vi "Total Nr instrument control to share.vi"() -> ()   [LabVIEW 2018]
panel:
  in  "MFC Max flow (ccm)":cluster{"MFC1":dbl, "MFC2":dbl}={"MFC1"=10000.0, "MFC2"=5000.0}
  out "NOx":cluster{"NO":dbl, "NO2":dbl, "NOx":dbl}(graph)
  out "NO2":dbl format="%#_13g"
  out "NOx":dbl format="%#_13g"
  out "NO":dbl format="%#_13g"
  out "MFC2":dbl format="%#_13g"
  in  "Cluster 2":cluster{"NOx":dbl, "NO":dbl, "NO2":dbl}
  out "Current reading (ppb)":cluster{"NO":dbl, "NOx":dbl, "NO2":dbl}
  in  "Start  Cal":bool
  out "Cal Running time (min)":sgl format="%#_3g"
  in  "read names":T1={"MFC1"="AIN0", "MFC2"="AIN1", "NO"="AIN2", "NOx"="AIN3", "NO2"="AIN5"}
  in  "write names":cluster{"MFC1":string, "MFC2":string}={"MFC1"="TDAC0", "MFC2"="TDAC1"}
  out "MFC flow (ccm)":cluster{"MFC1":dbl, "MFC2":dbl}
  in  "MFC setpoint (ccm)":cluster{"MFC1":dbl, "MFC2":dbl}={"MFC1"=1000.0, "MFC2"=0.0}
  out "valve 4":bool
  out "V4 loop no.":i32
  out "4":dbl
  in  "DIO names":T2={"DIO1"="EIO0", "DIO2"="EIO1", "DIO3"="EIO2", "DIO4"="EIO3", "DIO5"="EIO4", "DIO6"="EIO5"}
  out "Denuder\nTotal Nr":bool
  out "V3 loop no.":i32
  out "3":dbl
  out "Device Temp (K)":dbl[](array[numeric]) format="%.6f"
  in  "Valve switch":T3
  out "ConnectionType Out":i32
  out "DeviceType Out\n7 = T7":i32
  in  "Identifier":string="LJM_idANY"
  in  "ConnectionType":string="LJM_ctANY"
  in  "DeviceType":string="LJM_dtANY"
  out "Error String":string
  out "error out":errorcluster
  out "Total running \ntime (min)":dbl format="%#_3g"
  out "?":cluster{"1":dbl, dbl, dbl}(graph)
  out "1":dbl format="%#_13g"
  in  "Time interval (min)":T4={"Inlet HONO/Total Nr\nValve 1 "=10.0, "HONO/Nox\nValve 2"=5.0, "Total Nr Gas/NH3\nValve 3"=5.0, "valve 5"=1.0, "valve 6"=1.0, "valve 4"=1.0}
  out "2":dbl
  out "V1 loop no.":i32
  out "Total Nr\nNOx":bool
  out "NOx\nDenuder":bool
  out "V2 loop no.":i32
  in  "Stop":bool
  # "Total Reactive Nitrogen Instrument Control Panel"
  # "Measurement Valve State"
  # "NOx"
  # "Calibration"
  # "Diagnostics"
  # "MFC control"
  # "Note MFC control independent of valve control"
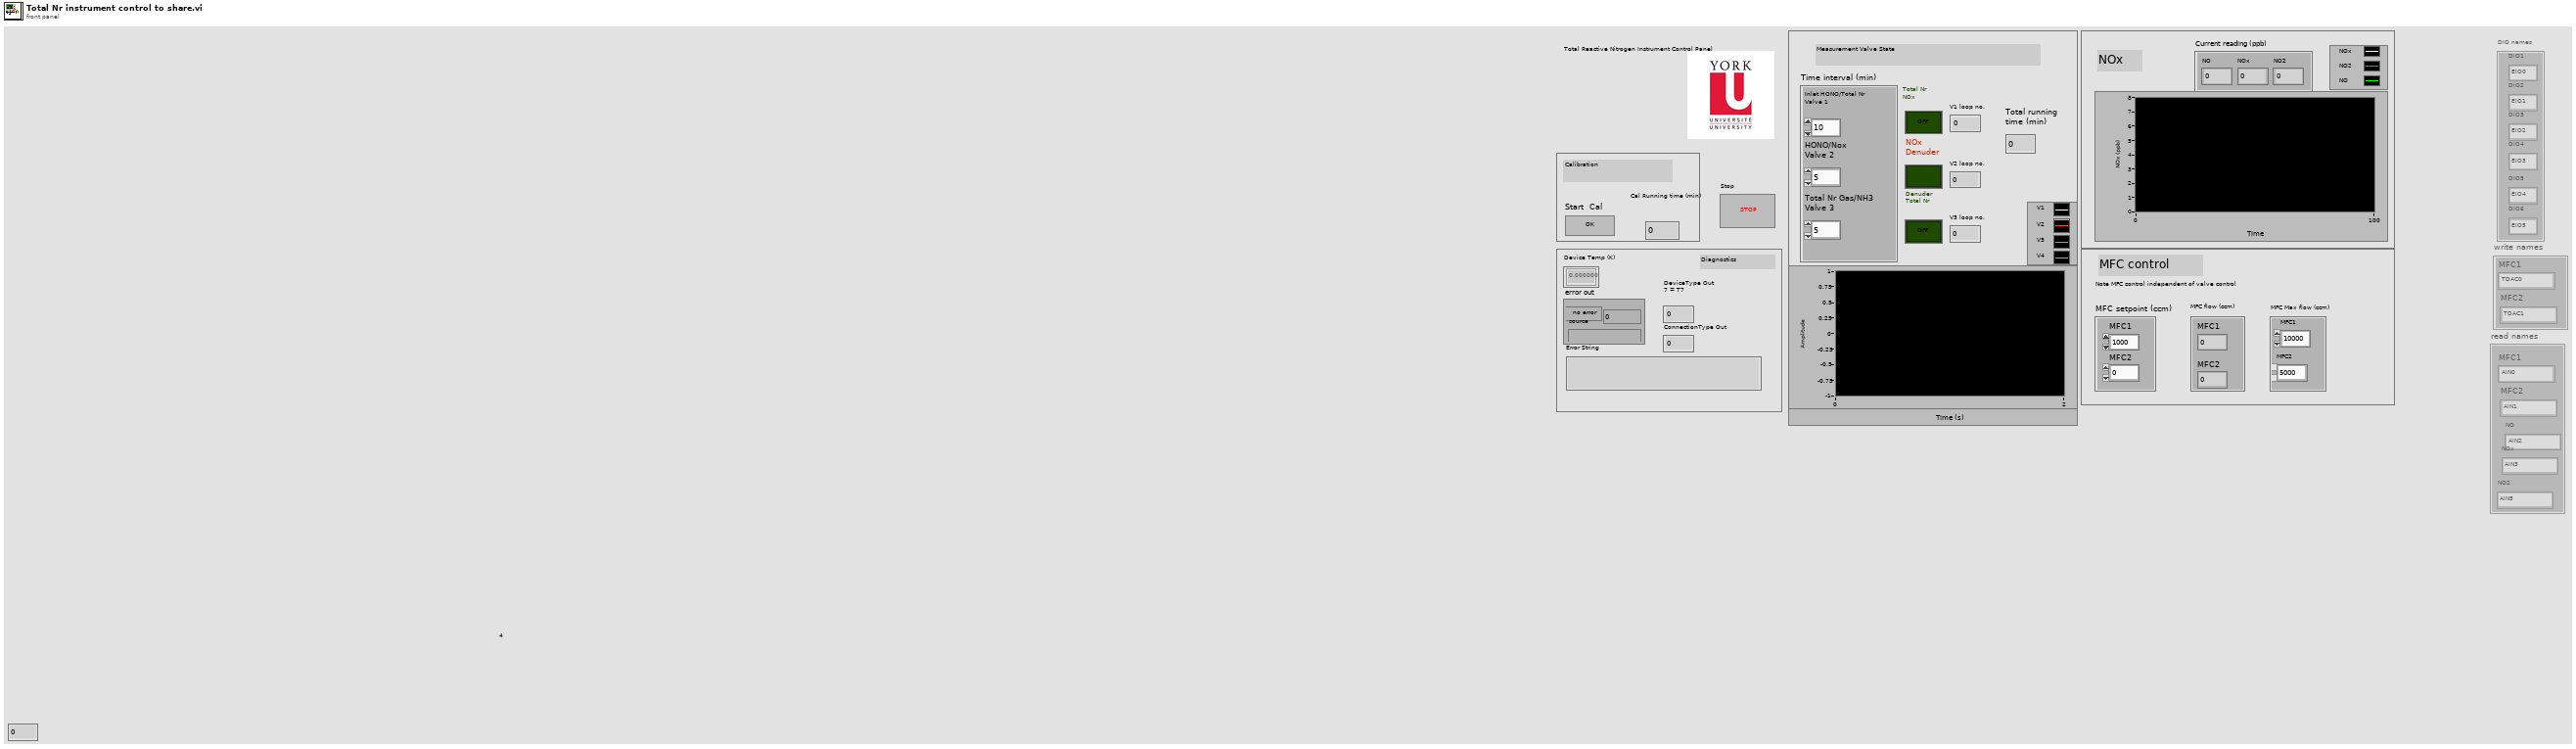
[diagram p1: front panel]
types:
  T1 = cluster{"MFC1":string, "MFC2":string, "NO":string, "NOx":string, "NO2":string}
  T2 = cluster{"DIO1":string, "DIO2":string, "DIO3":string, "DIO4":string, "DIO5":string, "DIO6":string}
  T3 = cluster{"S1":bool, "S2":bool, "S3":bool, "S4":bool, "S5":bool, "S6":bool, "S7":bool, "S8":bool, "S9":bool, "S10":bool, "S11":bool, "S12":bool}
  T4 = cluster{"Inlet HONO/Total Nr\nValve 1 ":dbl, "HONO/Nox\nValve 2":dbl, "Total Nr Gas/NH3\nValve 3":dbl, "valve 5":dbl, "valve 6":dbl, "valve 4":dbl}
  T5 = enum16{"open", "replace", "create", "open or create", "replace or create", "replace or create with confirmation"}
  T6 = cluster{"second":i32, "minute":i32, "hour":i32, "day of month":i32, "month":i32, "year":i32, "day of week":i32, "day of year":i32, "is DST":i32}
  T7 = cluster{"1":dbl, "2":dbl, "3":dbl, "4":dbl, "MFC2":dbl, "NO":dbl, "NO2":dbl, "NOx":dbl}
  T8 = cluster{"1":string, "2":string, "3":string, "4":string, "MFC2":string, "NO":string, "NO2":string, "NOx":string}
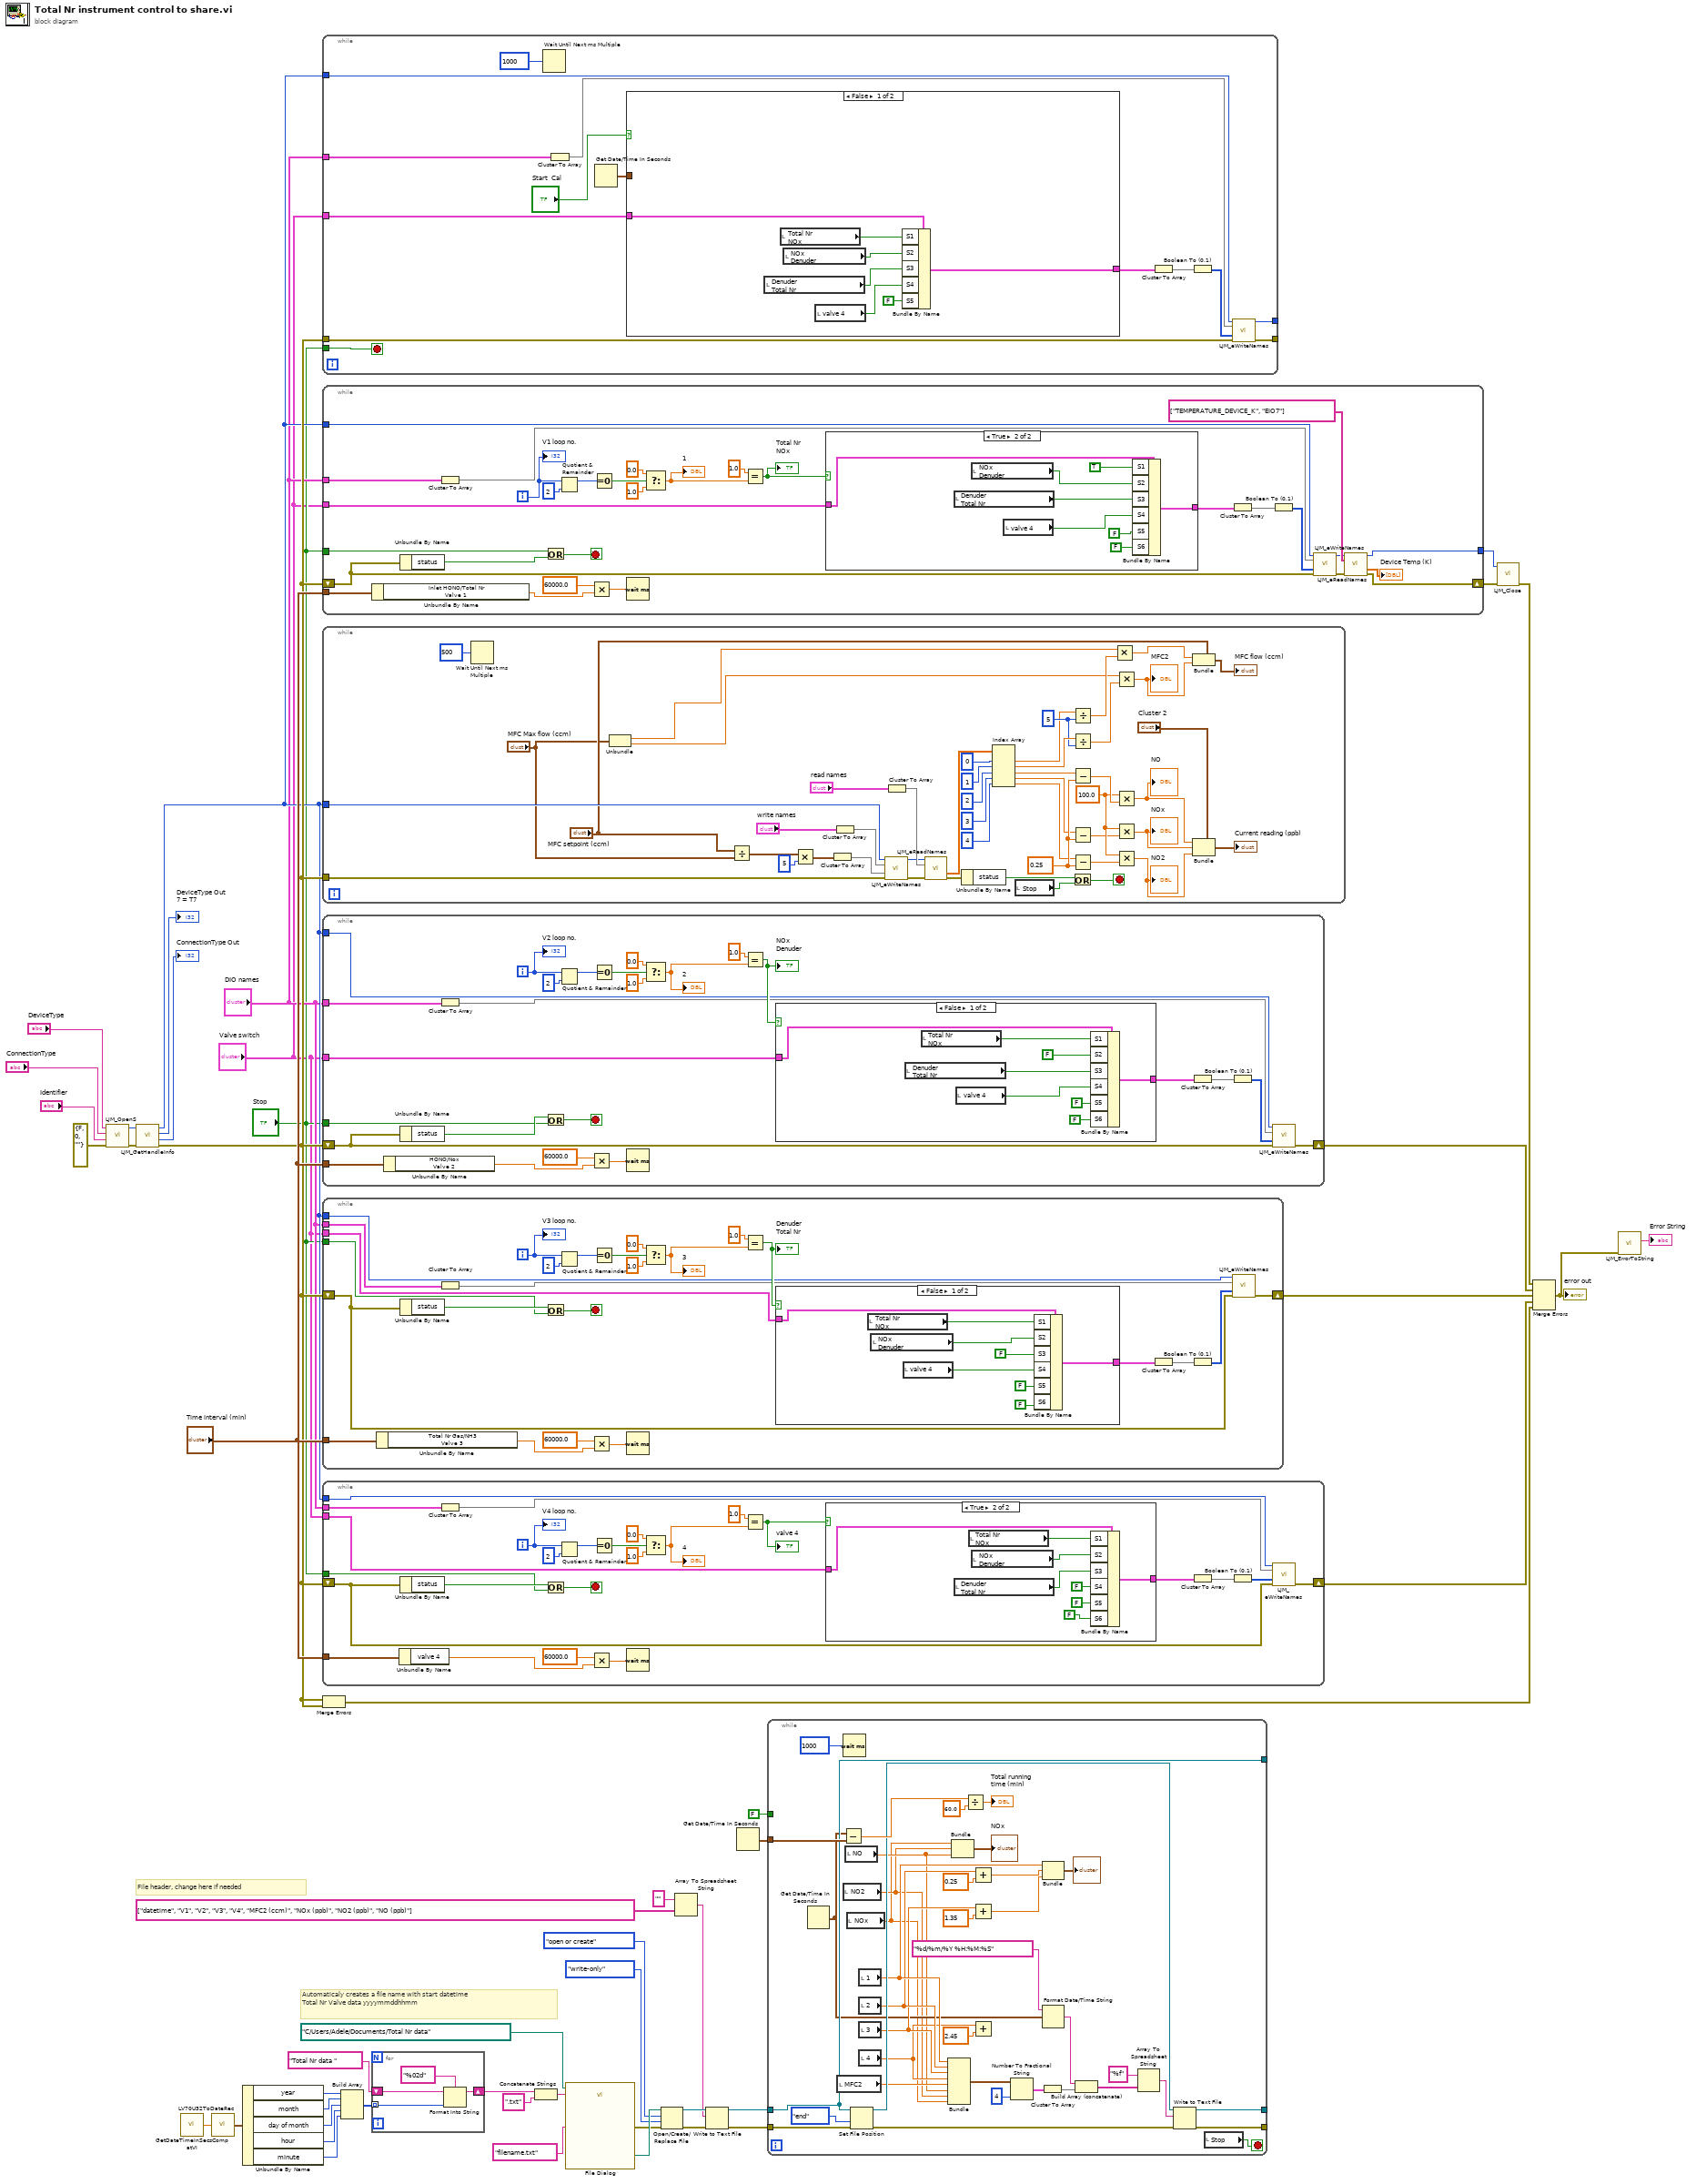
[diagram p0: block diagram]
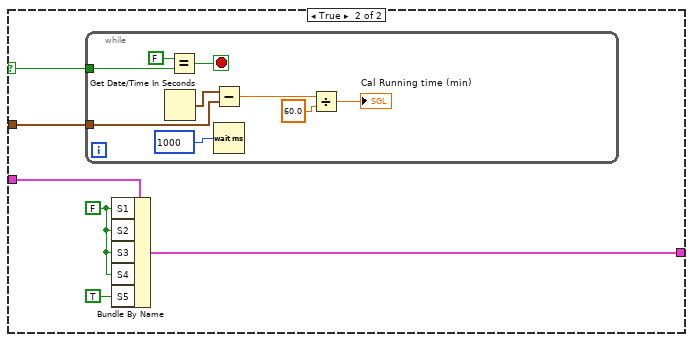
[diagram p2: hidden frame]
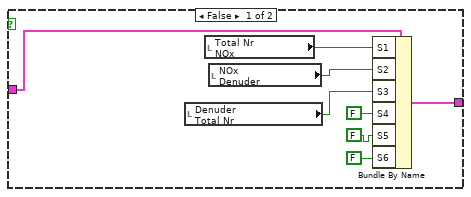
[diagram p3: hidden frame]
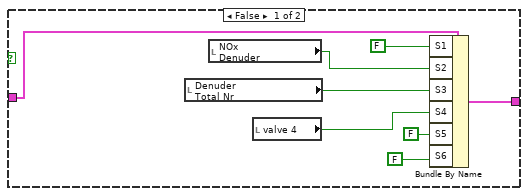
[diagram p4: hidden frame]
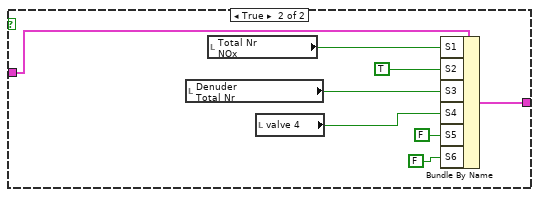
[diagram p5: hidden frame]
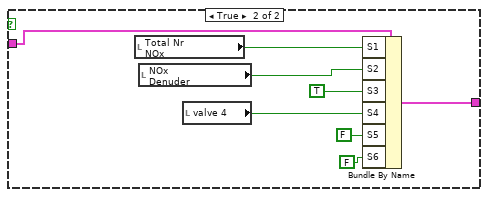
[diagram p6: hidden frame]
diagram:
  # "File header, change here if needed"
  # "Automaticaly creates a file name with start datetime\nTotal Nr Valve data yyyymmddhhmm"
  n1 = call "LJM_OpenS.vi"("error in"=errorcluster {"status"=FALSE, "code"=0, "source"=""} ("error in (no error)"), "Identifier"="Identifier", "ConnectionType"="ConnectionType", "DeviceType"="DeviceType") -> ("error out"=w47:errorcluster, "Handle"=w46:i32)  [unwired: 6 in]
  n2 = call "LJM_GetHandleInfo.vi"("error in"=w47, "Handle In"=w46) -> ("error out"=w5:errorcluster, "ConnectionType"=→"ConnectionType Out":i32, "DeviceType"=→"DeviceType Out\n7 = T7":i32, "Handle Out"=w4:i32)  [unwired: 2 in, 4 out]
  n3 = call <vilib>:"GetDateTimeInSecsCompatVI.vi"() -> ("double precision float"=w25:dbl)  [unwired: 1 in]
  n4 = call <vilib>:"LV70U32ToDateRec.vi"("Time"=w25) -> ("date time rec"=w33:T6)
  n5 = Unbundle By Name(w33) -> ("year"=w32:i32, "month"=w31:i32, "day of month"=w30:i32, "hour"=w29:i32, "minute"=w28:i32)
  n6 = while {
    tunnel: w4 -> [w61]
    tunnel: w5 -> [w60]
    tunnel: [w59] -> _
    tunnel: [w58] -> _
    tunnel: "DIO names" -> [w57]
    tunnel: "Stop" -> [w51]
    tunnel: "Valve switch" -> [w55]
    stop <- w51 stop-if-true
    n7 = Wait Until Next ms Multiple(millisecond multiple=1000 ("Interval [ms]")) -> ()  [unwired: 1 out]
    n8 = Cluster To Array(cluster=w57) -> (array=w56:string[])
    n9 = Get Date/Time In Seconds() -> (seconds since 1Jan1904=w52:timestamp)
    n10 = case shown="False" "Start  Cal" {
      selector: "Start  Cal" -> [_ w72]
      tunnel: w55 -> [w70 w77]
      tunnel: [w69 w76] -> w54
      tunnel: w52 -> [_ w75]
      frame False {
        n11 = local read "Denuder\nTotal Nr"() -> (w66:bool)
        n12 = local read "Total Nr\nNOx"() -> (w65:bool)
        n13 = local read "NOx\nDenuder"() -> (w68:bool)
        n14 = local read "valve 4"() -> (w67:bool)
        n15 = Bundle By Name(cluster=w70, "S1"=w65, "S2"=w68, "S3"=w66, "S4"=w67, "S5"=FALSE) -> (w69:T3)
      }
      frame True {
        w74 = FALSE
        n16 = while {
          tunnel: w75 -> [w86]
          tunnel: w72 -> [w80]
          stop <- w78 stop-if-true
          n17 = Get Date/Time In Seconds() -> (seconds since 1Jan1904=w85:timestamp)
          n18 = Equal?(x=FALSE, y=w80) -> (x = y?=w78:bool)
          n19 = Subtract(x=w85, y=w86) -> (x-y=w82:dbl)
          n20 = Wait (ms)(milliseconds to wait=1000) -> ()  [unwired: 1 out]
          n21 = Divide(x=w82, y=60.0) -> (x/y=→"Cal Running time (min)":dbl)
        }
        n22 = Bundle By Name(cluster=w77, "S1"=w74, "S2"=w74, "S3"=w74, "S4"=w74, "S5"=TRUE) -> (w76:T3)
      }
    }
    n23 = Cluster To Array(cluster=w54) -> (array=w62:bool[])
    n24 = Boolean To (0,1)(Boolean=w62) -> (0, 1=w63:i16[])
    n25 = call "LJM_eWriteNames.vi"("Handle In"=w61, "aNames"=w56, "aValuesIn"=w63, "error in"=w60) -> ("Handle Out"=w58:i32, "error out"=w59:errorcluster)  [unwired: 9 in, 1 out]
  }
  n26 = while {
    tunnel: "Stop" -> [w110]
    tunnel: "Time interval (min)" -> [w116]
    shift-right: [w91] -> w11
    shift-left: w5 -> [w112]
    tunnel: [w92] -> w10
    tunnel: w4 -> [w90]
    tunnel: "DIO names" -> [w87]
    tunnel: "Valve switch" -> [w88]
    i -> [w100]
    stop <- w109 stop-if-true
    n27 = Unbundle By Name(w116) -> ("Inlet HONO/Total Nr\nValve 1"=w96:dbl)
    n28 = Unbundle By Name(w112) -> ("status"=w111:bool)
    n29 = Cluster To Array(cluster=w87) -> (array=w89:string[])
    n30 = Or(x=w110, y=w111) -> (x .or. y?=w109:bool)
    n31 = Quotient & Remainder(x=w100, y=2) -> (x-y*floor(x/y)=w103:i32)  [unwired: 1 out]
    n32 = Multiply(x=60000.0, y=w96) -> (x*y=w97:dbl)
    n33 = Equal To 0?(x=w103) -> (x = 0?=w104:bool)
    n34 = Wait (ms)(milliseconds to wait=w97) -> ()  [unwired: 1 out]
    n35 = Select(t=0.0, s=w104, f=1.0) -> (s? t:f=w94:dbl)
    "1" <- w94
    n36 = Equal?(x=1.0, y=w94) -> (x = y?=w93:bool)
    "Total Nr\nNOx" <- w93
    n37 = case shown="True" w93 {
      tunnel: w88 -> [w124 w132]
      tunnel: [w123 w130] -> w115
      frame False {
        n38 = local read "Denuder\nTotal Nr"() -> (w120:bool)
        n39 = local read "NOx\nDenuder"() -> (w121:bool)
        n40 = local read "valve 4"() -> (w119:bool)
        n41 = Bundle By Name(cluster=w124, "S1"=FALSE, "S2"=w121, "S3"=w120, "S4"=w119, "S5"=FALSE, "S6"=FALSE) -> (w123:T3)
      }
      frame True {
        n42 = local read "Denuder\nTotal Nr"() -> (w128:bool)
        n43 = local read "NOx\nDenuder"() -> (w129:bool)
        n44 = local read "valve 4"() -> (w127:bool)
        n45 = Bundle By Name(cluster=w132, "S1"=TRUE, "S2"=w129, "S3"=w128, "S4"=w127, "S5"=FALSE, "S6"=FALSE) -> (w130:T3)
      }
    }
    n46 = Cluster To Array(cluster=w115) -> (array=w114:bool[])
    n47 = Boolean To (0,1)(Boolean=w114) -> (0, 1=w113:i16[])
    n48 = call "LJM_eWriteNames.vi"("Handle In"=w90, "aNames"=w89, "aValuesIn"=w113, "error in"=w112) -> ("Handle Out"=w105:i32, "error out"=w106:errorcluster)  [unwired: 9 in, 1 out]
    n49 = call "LJM_eReadNames.vi"("Handle In"=w105, "aNames"=string[] ["TEMPERATURE_DEVICE_K", "EIO7"] ("Read Temp 2"), "error in"=w106) -> ("Handle Out"=w92:i32, "aValuesOut"=→"Device Temp (K)":dbl[], "error out"=w91:errorcluster)  [unwired: 9 in, 1 out]
    "V1 loop no." <- w100
  }
  n50 = while {
    tunnel: w5 -> [w178]
    tunnel: w4 -> [w177]
    stop <- w174 stop-if-true
    w145 = 100.0
    w149 = 0.25
    w158 = 5
    n51 = Wait Until Next ms Multiple(millisecond multiple=500) -> ()  [unwired: 1 out]
    n52 = Unbundle("MFC Max flow (ccm)") -> ("MFC1"=w136:dbl, "MFC2"=w135:dbl)
    n53 = Divide(x="MFC setpoint (ccm)", y="MFC Max flow (ccm)") -> (x/y=w173:cluster{"MFC1":dbl, "MFC2":dbl})
    n54 = Multiply(x=w173, y=5) -> (x*y=w172:cluster{"MFC1":dbl, "MFC2":dbl})
    n55 = Cluster To Array(cluster=w172) -> (array=w171:dbl[])
    n56 = Cluster To Array(cluster="write names") -> (array=w169:string[])
    n57 = Cluster To Array(cluster="read names") -> (array=w168:string[])
    n58 = call "LJM_eWriteNames.vi"("Handle In"=w177, "aNames"=w169, "aValuesIn"=w171, "error in"=w178) -> ("Handle Out"=w166:i32, "error out"=w179:errorcluster)  [unwired: 9 in, 1 out]
    n59 = call "LJM_eReadNames.vi"("Handle In"=w166, "aNames"=w168, "error in"=w179) -> ("aValuesOut"=w163:dbl[], "error out"=w180:errorcluster)  [unwired: 9 in, 2 out]
    n60 = Unbundle By Name(w180) -> ("status"=w175:bool)
    n61 = Index Array(array=w163, index #1=0, index #2=1, index #3=2, index #4=3, index #5=4) -> (element #1=w134:dbl, element #2=w159:dbl, element #3=w133:dbl, element #4=w148:dbl, element #5=w147:dbl)
    n62 = local read "Stop"() -> (w176:bool)
    n63 = Divide(x=w134, y=w158) -> (x/y=w160:dbl)
    n64 = Divide(x=w159, y=w158) -> (x/y=w157:dbl)
    n65 = Subtract(x=w133, y=w149) -> (x-y=w150:dbl)
    n66 = Subtract(x=w148, y=w149) -> (x-y=w144:dbl)
    n67 = Subtract(x=w147, y=w149) -> (x-y=w146:dbl)
    n68 = Or(x=w175, y=w176) -> (x .or. y?=w174:bool)
    n69 = Multiply(x=w136, y=w160) -> (x*y=w156:dbl)
    n70 = Multiply(x=w135, y=w157) -> (x*y=w141:dbl)
    "MFC2" <- w141
    n71 = Multiply(x=w145, y=w150) -> (x*y=w140:dbl)
    "NO" <- w140
    n72 = Multiply(x=w145, y=w144) -> (x*y=w139:dbl)
    "NOx" <- w139
    n73 = Multiply(x=w145, y=w146) -> (x*y=w138:dbl)
    "NO2" <- w138
    n74 = Bundle(cluster="MFC setpoint (ccm)", "MFC1"=w156, "MFC2"=w141) -> (→"MFC flow (ccm)":cluster{"MFC1":dbl, "MFC2":dbl})
    n75 = Bundle(cluster="Cluster 2", "NOx"=w140, "NO"=w139, "NO2"=w138) -> (→"Current reading (ppb)":cluster{"NOx":dbl, "NO":dbl, "NO2":dbl})
  }
  n76 = while {
    tunnel: "Stop" -> [w200]
    tunnel: "Time interval (min)" -> [w204]
    tunnel: "Valve switch" -> [w182]
    shift-right: [w185] -> w13
    shift-left: w5 -> [w199]
    tunnel: w4 -> [w184]
    tunnel: "DIO names" -> [w181]
    i -> [w192]
    stop <- w198 stop-if-true
    n77 = Unbundle By Name(w204) -> ("HONO/Nox\nValve 2"=w186:dbl)
    n78 = Unbundle By Name(w199) -> ("status"=w201:bool)
    n79 = Cluster To Array(cluster=w181) -> (array=w183:string[])
    n80 = Or(x=w201, y=w200) -> (x .or. y?=w198:bool)
    n81 = Quotient & Remainder(x=w192, y=2) -> (x-y*floor(x/y)=w196:i32)  [unwired: 1 out]
    n82 = Multiply(x=60000.0, y=w186) -> (x*y=w187:dbl)
    n83 = Equal To 0?(x=w196) -> (x = 0?=w197:bool)
    n84 = Wait (ms)(milliseconds to wait=w187) -> ()  [unwired: 1 out]
    n85 = Select(t=0.0, s=w197, f=1.0) -> (s? t:f=w190:dbl)
    "2" <- w190
    n86 = Equal?(x=1.0, y=w190) -> (x = y?=w189:bool)
    "NOx\nDenuder" <- w189
    n87 = case shown="False" w189 {
      tunnel: w182 -> [w213 w221]
      tunnel: [w212 w220] -> w205
      frame False {
        n88 = local read "Denuder\nTotal Nr"() -> (w210:bool)
        n89 = local read "Total Nr\nNOx"() -> (w209:bool)
        n90 = local read "valve 4"() -> (w208:bool)
        n91 = Bundle By Name(cluster=w213, "S1"=w209, "S2"=FALSE, "S3"=w210, "S4"=w208, "S5"=FALSE, "S6"=FALSE) -> (w212:T3)
      }
      frame True {
        n92 = local read "Denuder\nTotal Nr"() -> (w217:bool)
        n93 = local read "Total Nr\nNOx"() -> (w219:bool)
        n94 = local read "valve 4"() -> (w216:bool)
        n95 = Bundle By Name(cluster=w221, "S1"=w219, "S2"=TRUE, "S3"=w217, "S4"=w216, "S5"=FALSE, "S6"=FALSE) -> (w220:T3)
      }
    }
    n96 = Cluster To Array(cluster=w205) -> (array=w203:bool[])
    n97 = Boolean To (0,1)(Boolean=w203) -> (0, 1=w202:i16[])
    n98 = call "LJM_eWriteNames.vi"("Handle In"=w184, "aNames"=w183, "aValuesIn"=w202, "error in"=w199) -> ("error out"=w185:errorcluster)  [unwired: 9 in, 2 out]
    "V2 loop no." <- w192
  }
  n99 = while {
    tunnel: "Stop" -> [w241]
    tunnel: "Time interval (min)" -> [w245]
    tunnel: "Valve switch" -> [w223]
    shift-right: [w226] -> w9
    shift-left: w5 -> [w240]
    tunnel: w4 -> [w225]
    tunnel: "DIO names" -> [w222]
    i -> [w233]
    stop <- w239 stop-if-true
    n100 = Unbundle By Name(w245) -> ("Total Nr Gas/NH3\nValve 3"=w227:dbl)
    n101 = Unbundle By Name(w240) -> ("status"=w242:bool)
    n102 = Cluster To Array(cluster=w222) -> (array=w224:string[])
    n103 = Or(x=w242, y=w241) -> (x .or. y?=w239:bool)
    n104 = Quotient & Remainder(x=w233, y=2) -> (x-y*floor(x/y)=w237:i32)  [unwired: 1 out]
    n105 = Multiply(x=60000.0, y=w227) -> (x*y=w228:dbl)
    n106 = Equal To 0?(x=w237) -> (x = 0?=w238:bool)
    n107 = Wait (ms)(milliseconds to wait=w228) -> ()  [unwired: 1 out]
    n108 = Select(t=0.0, s=w238, f=1.0) -> (s? t:f=w231:dbl)
    "3" <- w231
    n109 = Equal?(x=1.0, y=w231) -> (x = y?=w230:bool)
    "Denuder\nTotal Nr" <- w230
    n110 = case shown="False" w230 {
      tunnel: w223 -> [w254 w262]
      tunnel: [w253 w261] -> w246
      frame False {
        n111 = local read "Total Nr\nNOx"() -> (w251:bool)
        n112 = local read "NOx\nDenuder"() -> (w250:bool)
        n113 = local read "valve 4"() -> (w249:bool)
        n114 = Bundle By Name(cluster=w254, "S1"=w251, "S2"=w250, "S3"=FALSE, "S4"=w249, "S5"=FALSE, "S6"=FALSE) -> (w253:T3)
      }
      frame True {
        n115 = local read "Total Nr\nNOx"() -> (w259:bool)
        n116 = local read "NOx\nDenuder"() -> (w258:bool)
        n117 = local read "valve 4"() -> (w257:bool)
        n118 = Bundle By Name(cluster=w262, "S1"=w259, "S2"=w258, "S3"=TRUE, "S4"=w257, "S5"=FALSE, "S6"=FALSE) -> (w261:T3)
      }
    }
    n119 = Cluster To Array(cluster=w246) -> (array=w244:bool[])
    n120 = Boolean To (0,1)(Boolean=w244) -> (0, 1=w243:i16[])
    n121 = call "LJM_eWriteNames.vi"("Handle In"=w225, "aNames"=w224, "aValuesIn"=w243, "error in"=w240) -> ("error out"=w226:errorcluster)  [unwired: 9 in, 2 out]
    "V3 loop no." <- w233
  }
  n122 = while {
    tunnel: "Stop" -> [w282]
    tunnel: "Time interval (min)" -> [w286]
    tunnel: "Valve switch" -> [w264]
    shift-right: [w267] -> w8
    shift-left: w5 -> [w281]
    tunnel: w4 -> [w266]
    tunnel: "DIO names" -> [w263]
    i -> [w274]
    stop <- w280 stop-if-true
    n123 = Unbundle By Name(w286) -> ("valve 4"=w268:dbl)
    n124 = Unbundle By Name(w281) -> ("status"=w283:bool)
    n125 = Cluster To Array(cluster=w263) -> (array=w265:string[])
    n126 = Or(x=w283, y=w282) -> (x .or. y?=w280:bool)
    n127 = Quotient & Remainder(x=w274, y=2) -> (x-y*floor(x/y)=w278:i32)  [unwired: 1 out]
    n128 = Multiply(x=60000.0, y=w268) -> (x*y=w269:dbl)
    n129 = Equal To 0?(x=w278) -> (x = 0?=w279:bool)
    n130 = Wait (ms)(milliseconds to wait=w269) -> ()  [unwired: 1 out]
    n131 = Select(t=0.0, s=w279, f=1.0) -> (s? t:f=w272:dbl)
    "4" <- w272
    n132 = Equal?(x=1.0, y=w272) -> (x = y?=w271:bool)
    "valve 4" <- w271
    n133 = case shown="True" w271 {
      tunnel: w264 -> [w295 w303]
      tunnel: [w294 w302] -> w287
      frame False {
        n134 = local read "Denuder\nTotal Nr"() -> (w291:bool)
        n135 = local read "Total Nr\nNOx"() -> (w293:bool)
        n136 = local read "NOx\nDenuder"() -> (w292:bool)
        n137 = Bundle By Name(cluster=w295, "S1"=w293, "S2"=w292, "S3"=w291, "S4"=FALSE, "S5"=FALSE, "S6"=FALSE) -> (w294:T3)
      }
      frame True {
        n138 = local read "Denuder\nTotal Nr"() -> (w298:bool)
        n139 = local read "Total Nr\nNOx"() -> (w301:bool)
        n140 = local read "NOx\nDenuder"() -> (w299:bool)
        n141 = Bundle By Name(cluster=w303, "S1"=w301, "S2"=w299, "S3"=w298, "S4"=FALSE, "S5"=FALSE, "S6"=FALSE) -> (w302:T3)
      }
    }
    n142 = Cluster To Array(cluster=w287) -> (array=w285:bool[])
    n143 = Boolean To (0,1)(Boolean=w285) -> (0, 1=w284:i16[])
    n144 = call "LJM_eWriteNames.vi"("Handle In"=w266, "aNames"=w265, "aValuesIn"=w284, "error in"=w281) -> ("error out"=w267:errorcluster)  [unwired: 9 in, 2 out]
    "V4 loop no." <- w274
  }
  n145 = Merge Errors(w5, w5) -> (w7:errorcluster)
  n146 = Build Array(w32, w31, w30, w29, w28) -> (w27:i32[])
  n147 = for {
    tunnel: w27 -> [w307] mode=indexing
    shift-right: [w306] -> w23
    shift-left: "Total Nr data " ("PreString") -> [w305]
    n148 = Format Into String(format string="%02d", initial string=w305, w307) -> (resulting string=w306:string)  [unwired: 1 in, 1 out]
  }
  n149 = Concatenate Strings(w23, ".txt" ("Poststring")) -> (w22:string)
  n150 = call "File Dialog"("start path"=path "C:/Users/Adele/Documents/Total Nr data", "prompt"="filename.txt", "default name"=w22) -> ("selected path"=w39:path, "error out"=w38:errorcluster)  [unwired: 9 in, 2 out]
  n151 = Open/Create/Replace File(file path (use dialog)=w39, error in=w38, operation (0:open)=T5."open or create", access (0:read/write)=enum16{"read/write", "read-only", "write-only"}."write-only") -> (refnum out=w20:refnum<file>, error out=w15:errorcluster)  [unwired: 2 in, 1 out]
  n152 = Array To Spreadsheet String(array=string[] ["datetime", "V1", "V2", "V3", "V4", "MFC2 (ccm)", "NOx (ppb)", "NO2 (ppb)", "NO (ppb)"], 3:"") -> (spreadsheet string=w16:string)  [unwired: 1 in]
  n153 = Write to Text File(file (use dialog)=w20, text=w16, error in=w15) -> (refnum out=w19:refnum<file>, error out=w14:errorcluster)  [unwired: 1 in, 1 out]
  n154 = Get Date/Time In Seconds() -> (seconds since 1Jan1904=w50:timestamp)
  n155 = while {
    tunnel: w50 -> [w343]
    tunnel: FALSE -> [_]
    tunnel: w14 -> [w333]
    tunnel: [w316] -> _
    tunnel: [w323] -> _
    tunnel: [w317] -> _
    tunnel: w19 -> [w316]
    stop <- w345 stop-if-true
    n156 = Get Date/Time In Seconds() -> (seconds since 1Jan1904=w315:timestamp)
    n157 = local read "MFC2"() -> (w312:dbl)
    n158 = Subtract(x=w315, y=w343) -> (x-y=w341:dbl)
    n159 = Wait (ms)(milliseconds to wait=1000) -> ()  [unwired: 1 out]
    n160 = local read "NO2"() -> (w309:dbl)
    n161 = local read "NO"() -> (w310:dbl)
    n162 = local read "NOx"() -> (w308:dbl)
    n163 = Set File Position(refnum=w316, from (0:start)=enum16{"start", "end", "current"}."end", error in=w333) -> (refnum out=w325:refnum<file>, error out=w324:errorcluster)  [unwired: 1 in]
    n164 = local read "1"() -> (w322:dbl)
    n165 = local read "2"() -> (w321:dbl)
    n166 = local read "3"() -> (w320:dbl)
    n167 = local read "4"() -> (w319:dbl)
    n168 = Bundle("1"=w322, "2"=w321, "3"=w320, "4"=w319, "MFC2"=w312, "NO"=w310, "NO2"=w309, "NOx"=w308) -> (w318:T7)  [unwired: 1 in]
    n169 = Bundle("NOx"=w308, "NO2"=w309, "NO"=w310) -> (→"NOx":cluster{"NOx":dbl, "NO2":dbl, "NO":dbl})  [unwired: 1 in]
    n170 = Divide(x=w341, y=60.0) -> (x/y=→"Total running \ntime (min)":dbl)
    n171 = Add(x=w321, y=0.25) -> (x+y=w336:dbl)
    n172 = Add(x=w320, y=1.35) -> (x+y=w338:dbl)
    n173 = Add(x=w319, y=2.45) -> ()  [unwired: 1 out]
    n174 = Number To Fractional String(number=w318, precision (6)=4) -> (F-format string=w327:T8)  [unwired: 2 in]
    n175 = Cluster To Array(cluster=w327) -> (array=w326:string[])
    n176 = Bundle("1"=w322, w336, w338) -> (→"?":cluster{"1":dbl, dbl, dbl})  [unwired: 1 in]
    n177 = Format Date/Time String(time format string (%c)="%d/%m/%Y %H:%M:%S", seconds (now)=w315) -> (date/time string=w313:string)  [unwired: 1 in]
    n178 = Build Array (concatenate)(w313, w326) -> (w330:string[])
    n179 = Array To Spreadsheet String(array=w330, 3:"%f" ("format string")) -> (spreadsheet string=w329:string)  [unwired: 1 in]
    n180 = Write to Text File(file (use dialog)=w325, text=w329, error in=w324) -> (refnum out=w323:refnum<file>, error out=w317:errorcluster)  [unwired: 1 in, 1 out]
    n181 = local read "Stop"() -> (w345:bool)
  }
  n182 = call "LJM_Close.vi"("error in"=w11, "Handle"=w10) -> ("error out"=w12:errorcluster)  [unwired: 9 in]
  n183 = Merge Errors(w12, w13, w9, w8, w7) -> (w40:errorcluster)
  "error out" <- w40
  n184 = call "LJM_ErrorToString.vi"("error in"=w40) -> ("String"=→"Error String":string)  [unwired: 10 in]
